vi "TalkToCVServer.vi"() -> ()   [LabVIEW 2019]
panel:
  out "Streaming":T1
  in  "Stop":bool
  out "Commands":T2(array[cluster])=[{"Info"={"version"="1.0", "Code"=200, "type"="text/html", "length"=-1}, "Header"="HTTP/1.0 200 OK\r\nServer: BaseHTTP/0.6 Python/3.7.2\r\nDate: Mon, 07 Dec 2020 21:12:43 GMT\r\nContent-type: text/html\r\n\r\n", "Body"="<html><head><title>Rogers Camera Code</title></head>\n                        <body><p>Rogers Camera  (192.168.86.35)<br>Camera Status: not connected</p>\n                        <a href = \"http://192.168.86.35:8000/settings\">Current Settings</a><br>\n                        <a href = \"http://192.168.86.35:8000/init\">Initialize Camera</a><br>\n                        <a href = \"http://192.168.86.35:8000/snap\">Snap an Image</a><br>\n                        <a href = \"http://192.168.86.35:8000/grab\">Stream Images</a><br>\n                        <a href = \"http://192.168.86.35:8000/close\">Close Camera Connection</a><br><br><br>\n                        <form action=\"/settings\"> \n                        <label for=\"camera\">Camera:</label>  \n                        <input type=\"number\" id=\"camera\" name=\"camera\" value=\"1\"><br> \n                        <label for=\"scale\">Scale Percent:</label>  \n                        <input type=\"number\" id=\"scale\" name=\"scale\" value=\"20\"><br>  \n                        <label for=\"rotate\">Orientation:</label> \n                        <select name=\"rotate\" id=\"rotate\" value=\"-1\"> \n                          <option value=\"-1\">no rotation</option> \n                          <option value=\"0\">90 CW</option> \n                          <option value=\"1\">180</option> \n                          <option value=\"2\">90 CCW</option> \n                        </select> <br><br>\n                        <input type=\"submit\" value=\"Update\">  \n                    </form><hr><p>Executing command: /</p></body></html>\r\n", "2D Picture"=bytes[494]}, {"Info"={"version"="1.0", "Code"=200, "type"="text/html", "length"=-1}, "Header"="HTTP/1.0 200 OK\r\nServer: BaseHTTP/0.6 Python/3.7.2\r\nDate: Mon, 07 Dec 2020 21:12:44 GMT\r\nContent-type: text/html\r\n\r\n", "Body"="<html><head><title>Rogers Camera Code</title></head>\n                        <body><p>Rogers Camera  (192.168.86.35)<br>Camera Status: not connected</p>\n                        <a href = \"http://192.168.86.35:8000/settings\">Current Settings</a><br>\n                        <a href = \"http://192.168.86.35:8000/init\">Initialize Camera</a><br>\n                        <a href = \"http://192.168.86.35:8000/snap\">Snap an Image</a><br>\n                        <a href = \"http://192.168.86.35:8000/grab\">Stream Images</a><br>\n                        <a href = \"http://192.168.86.35:8000/close\">Close Camera Connection</a><br><br><br>\n                        <form action=\"/settings\"> \n                        <label for=\"camera\">Camera:</label>  \n                        <input type=\"number\" id=\"camera\" name=\"camera\" value=\"1\"><br> \n                        <label for=\"scale\">Scale Percent:</label>  \n                        <input type=\"number\" id=\"scale\" name=\"scale\" value=\"40\"><br>  \n                        <label for=\"rotate\">Orientation:</label> \n                        <select name=\"rotate\" id=\"rotate\" value=\"-1\"> \n                          <option value=\"-1\">no rotation</option> \n                          <option value=\"0\">90 CW</option> \n                          <option value=\"1\">180</option> \n                          <option value=\"2\">90 CCW</option> \n                        </select> <br><br>\n                        <input type=\"submit\" value=\"Update\">  \n                    </form><hr><p>Executing command: /settings?camera=1&rotation=-1&scale=40</p>Settings:<br>Camera = 1<br>scaling = 40<br>Rotation = -1</body></html>\r\n", "2D Picture"=bytes[580]}, {"Info"={"version"="1.0", "Code"=200, "type"="text/html", "length"=-1}, "Header"="HTTP/1.0 200 OK\r\nServer: BaseHTTP/0.6 Python/3.7.2\r\nDate: Mon, 07 Dec 2020 21:12:44 GMT\r\nContent-type: text/html\r\n\r\n", "Body"="<html><head><title>Rogers Camera Code</title></head>\n                        <body><p>Rogers Camera  (192.168.86.35)<br>Camera Status: connected</p>\n                        <a href = \"http://192.168.86.35:8000/settings\">Current Settings</a><br>\n                        <a href = \"http://192.168.86.35:8000/init\">Initialize Camera</a><br>\n                        <a href = \"http://192.168.86.35:8000/snap\">Snap an Image</a><br>\n                        <a href = \"http://192.168.86.35:8000/grab\">Stream Images</a><br>\n                        <a href = \"http://192.168.86.35:8000/close\">Close Camera Connection</a><br><br><br>\n                        <form action=\"/settings\"> \n                        <label for=\"camera\">Camera:</label>  \n                        <input type=\"number\" id=\"camera\" name=\"camera\" value=\"1\"><br> \n                        <label for=\"scale\">Scale Percent:</label>  \n                        <input type=\"number\" id=\"scale\" name=\"scale\" value=\"40\"><br>  \n                        <label for=\"rotate\">Orientation:</label> \n                        <select name=\"rotate\" id=\"rotate\" value=\"-1\"> \n                          <option value=\"-1\">no rotation</option> \n                          <option value=\"0\">90 CW</option> \n                          <option value=\"1\">180</option> \n                          <option value=\"2\">90 CCW</option> \n                        </select> <br><br>\n                        <input type=\"submit\" value=\"Update\">  \n                    </form><hr><p>Executing command: /init</p>initializing camera # 1</body></html>\r\n", "2D Picture"=bytes[518]}, {"Info"={"version"="1.0", "Code"=200, "type"="text/html", "length"=-1}, "Header"="HTTP/1.0 200 OK\r\nServer: BaseHTTP/0.6 Python/3.7.2\r\nDate: Mon, 07 Dec 2020 21:12:45 GMT\r\nContent-type: text/html\r\n\r\n", "Body"="<html><head><title>Rogers Camera Code</title></head>\n                        <body><p>Rogers Camera  (192.168.86.35)<br>Camera Status: connected</p>\n                        <a href = \"http://192.168.86.35:8000/settings\">Current Settings</a><br>\n                        <a href = \"http://192.168.86.35:8000/init\">Initialize Camera</a><br>\n                        <a href = \"http://192.168.86.35:8000/snap\">Snap an Image</a><br>\n                        <a href = \"http://192.168.86.35:8000/grab\">Stream Images</a><br>\n                        <a href = \"http://192.168.86.35:8000/close\">Close Camera Connection</a><br><br><br>\n                        <form action=\"/settings\"> \n                        <label for=\"camera\">Camera:</label>  \n                        <input type=\"number\" id=\"camera\" name=\"camera\" value=\"1\"><br> \n                        <label for=\"scale\">Scale Percent:</label>  \n                        <input type=\"number\" id=\"scale\" name=\"scale\" value=\"40\"><br>  \n                        <label for=\"rotate\">Orientation:</label> \n                        <select name=\"rotate\" id=\"rotate\" value=\"-1\"> \n                          <option value=\"-1\">no rotation</option> \n                          <option value=\"0\">90 CW</option> \n                          <option value=\"1\">180</option> \n                          <option value=\"2\">90 CCW</option> \n                        </select> <br><br>\n                        <input type=\"submit\" value=\"Update\">  \n                    </form><hr><p>Executing command: /snap</p>snapping from camera # 1<br><br><img src=\"http://192.168.86.35:8000/snap.jpg\"></body></html>\r\n", "2D Picture"=bytes[37460]}, {"Info"={"version"="1.0", "Code"=200, "type"="text/html", "length"=-1}, "Header"="HTTP/1.0 200 OK\r\nServer: BaseHTTP/0.6 Python/3.7.2\r\nDate: Mon, 07 Dec 2020 21:12:45 GMT\r\nContent-type: text/html\r\n\r\n", "Body"="<html><head><title>Rogers Camera Code</title></head>\n                        <body><p>Rogers Camera  (192.168.86.35)<br>Camera Status: connected</p>\n                        <a href = \"http://192.168.86.35:8000/settings\">Current Settings</a><br>\n                        <a href = \"http://192.168.86.35:8000/init\">Initialize Camera</a><br>\n                        <a href = \"http://192.168.86.35:8000/snap\">Snap an Image</a><br>\n                        <a href = \"http://192.168.86.35:8000/grab\">Stream Images</a><br>\n                        <a href = \"http://192.168.86.35:8000/close\">Close Camera Connection</a><br><br><br>\n                        <form action=\"/settings\"> \n                        <label for=\"camera\">Camera:</label>  \n                        <input type=\"number\" id=\"camera\" name=\"camera\" value=\"1\"><br> \n                        <label for=\"scale\">Scale Percent:</label>  \n                        <input type=\"number\" id=\"scale\" name=\"scale\" value=\"40\"><br>  \n                        <label for=\"rotate\">Orientation:</label> \n                        <select name=\"rotate\" id=\"rotate\" value=\"-1\"> \n                          <option value=\"-1\">no rotation</option> \n                          <option value=\"0\">90 CW</option> \n                          <option value=\"1\">180</option> \n                          <option value=\"2\">90 CCW</option> \n                        </select> <br><br>\n                        <input type=\"submit\" value=\"Update\">  \n                    </form><hr><p>Executing command: /bad</p>unsupported path</body></html>\r\n", "2D Picture"=bytes[510]}, {"Info"={"version"="1.0", "Code"=200, "type"="text/html", "length"=-1}, "Header"="HTTP/1.0 200 OK\r\nServer: BaseHTTP/0.6 Python/3.7.2\r\nDate: Mon, 07 Dec 2020 21:12:45 GMT\r\nContent-type: text/html\r\n\r\n", "Body"="<html><head><title>Rogers Camera Code</title></head>\n                        <body><p>Rogers Camera  (192.168.86.35)<br>Camera Status: connected</p>\n                        <a href = \"http://192.168.86.35:8000/settings\">Current Settings</a><br>\n                        <a href = \"http://192.168.86.35:8000/init\">Initialize Camera</a><br>\n                        <a href = \"http://192.168.86.35:8000/snap\">Snap an Image</a><br>\n                        <a href = \"http://192.168.86.35:8000/grab\">Stream Images</a><br>\n                        <a href = \"http://192.168.86.35:8000/close\">Close Camera Connection</a><br><br><br>\n                        <form action=\"/settings\"> \n                        <label for=\"camera\">Camera:</label>  \n                        <input type=\"number\" id=\"camera\" name=\"camera\" value=\"1\"><br> \n                        <label for=\"scale\">Scale Percent:</label>  \n                        <input type=\"number\" id=\"scale\" name=\"scale\" value=\"40\"><br>  \n                        <label for=\"rotate\">Orientation:</label> \n                        <select name=\"rotate\" id=\"rotate\" value=\"-1\"> \n                          <option value=\"-1\">no rotation</option> \n                          <option value=\"0\">90 CW</option> \n                          <option value=\"1\">180</option> \n                          <option value=\"2\">90 CCW</option> \n                        </select> <br><br>\n                        <input type=\"submit\" value=\"Update\">  \n                    </form><hr><p>Executing command: /settings</p>Settings:<br>Camera = 1<br>scaling = 40<br>Rotation = -1</body></html>\r\n", "2D Picture"=bytes[546]}, {"Info"={"version"="error", "Code"=0, "type"="image/jpeg", "length"=3460}, "Header"="--jpgboundary\r\nContent-type: image/jpeg\r\nContent-length: 3460\r\n\r\n", "Body"="ÿØÿà\u0000\u0010JFIF\u0000\u0001\u0001\u0000\u0000\u0001\u0000\u0001\u0000\u0000ÿÛ\u0000C\u0000\u0002\u0001\u0001\u0001\u0001\u0001\u0002\u0001\u0001\u0001\u0002\u0002\u0002\u0002\u0002\u0004\u0003\u0002\u0002\u0002\u0002\u0005\u0004\u0004\u0003\u0004\u0006\u0005\u0006\u0006\u0006\u0005\u0006\u0006\u0006\u0007\t\b\u0006\u0007\t\u0007\u0006\u0006\b\u000b\b\t\n\n\n\n\n\u0006\b\u000b\f\u000b\n\f\t\n\n\nÿÛ\u0000C\u0001\u0002\u0002\u0002\u0002\u0002\u0002\u0005\u0003\u0003\u0005\n\u0007\u0006\u0007\n\n\n\n\n\n\n\n\n\n\n\n\n\n\n\n\n\n\n\n\n\n\n\n\n\n\n\n\n\n\n\n\n\n\n\n\n\n\n\n\n\n\n\n\n\n\n\n\n\nÿÀ\u0000\u0011\b\u0000`\u0000\u0003\u0001\"\u0000\u0002\u0011\u0001\u0003\u0011\u0001ÿÄ\u0000\u001f\u0000\u0000\u0001\u0005\u0001\u0001\u0001\u0001\u0001\u0001\u0000\u0000\u0000\u0000\u0000\u0000\u0000\u0000\u0001\u0002\u0003\u0004\u0005\u0006\u0007\b\t\n\u000bÿÄ\u0000µ\u0010\u0000\u0002\u0001\u0003\u0003\u0002\u0004\u0003\u0005\u0005\u0004\u0004\u0000\u0000\u0001}\u0001\u0002\u0003\u0000\u0004\u0011\u0005\u0012!1A\u0006\u0013Qa\u0007\"q\u00142¡\b#B±Á\u0015RÑð$3br\t\n\u0016\u0017\u0018\u0019\u001a%&'()*456789:CDEFGHIJSTUVWXYZcdefghijstuvwxyz¢£¤¥¦§¨©ª²³´µ¶·¸¹ºÂÃÄÅÆÇÈÉÊÒÓÔÕÖ×ØÙÚáâãäåæçèéêñòóôõö÷øùúÿÄ\u0000\u001f\u0001\u0000\u0003\u0001\u0001\u0001\u0001\u0001\u0001\u0001\u0001\u0001\u0000\u0000\u0000\u0000\u0000\u0000\u0001\u0002\u0003\u0004\u0005\u0006\u0007\b\t\n\u000bÿÄ\u0000µ\u0011\u0000\u0002\u0001\u0002\u0004\u0004\u0003\u0004\u0007\u0005\u0004\u0004\u0000\u0001\u0002w\u0000\u0001\u0002\u0003\u0011\u0004\u0005!1\u0006\u0012AQ\u0007aq\u0013\"2\b\u0014B¡±Á\t#3Rð\u0015brÑ\n\u0016$4á%ñ\u0017\u0018\u0019\u001a&'()*56789:CDEFGHIJSTUVWXYZcdefghijstuvwxyz¢£¤¥¦§¨©ª²³´µ¶·¸¹ºÂÃÄÅÆÇÈÉÊÒÓÔÕÖ×ØÙÚâãäåæçèéê...", "2D Picture"=bytes[36894]}, {"Info"={"version"="1.0", "Code"=200, "type"="text/html", "length"=-1}, "Header"="HTTP/1.0 200 OK\r\nServer: BaseHTTP/0.6 Python/3.7.2\r\nDate: Mon, 07 Dec 2020 21:12:48 GMT\r\nContent-type: text/html\r\n\r\n", "Body"="<html><head><title>Rogers Camera Code</title></head>\n                        <body><p>Rogers Camera  (192.168.86.35)<br>Camera Status: not connected</p>\n                        <a href = \"http://192.168.86.35:8000/settings\">Current Settings</a><br>\n                        <a href = \"http://192.168.86.35:8000/init\">Initialize Camera</a><br>\n                        <a href = \"http://192.168.86.35:8000/snap\">Snap an Image</a><br>\n                        <a href = \"http://192.168.86.35:8000/grab\">Stream Images</a><br>\n                        <a href = \"http://192.168.86.35:8000/close\">Close Camera Connection</a><br><br><br>\n                        <form action=\"/settings\"> \n                        <label for=\"camera\">Camera:</label>  \n                        <input type=\"number\" id=\"camera\" name=\"camera\" value=\"1\"><br> \n                        <label for=\"scale\">Scale Percent:</label>  \n                        <input type=\"number\" id=\"scale\" name=\"scale\" value=\"40\"><br>  \n                        <label for=\"rotate\">Orientation:</label> \n                        <select name=\"rotate\" id=\"rotate\" value=\"-1\"> \n                          <option value=\"-1\">no rotation</option> \n                          <option value=\"0\">90 CW</option> \n                          <option value=\"1\">180</option> \n                          <option value=\"2\">90 CCW</option> \n                        </select> <br><br>\n                        <input type=\"submit\" value=\"Update\">  \n                    </form><hr><p>Executing command: /close</p>closing camera # 1</body></html>\r\n", "2D Picture"=bytes[518]}]
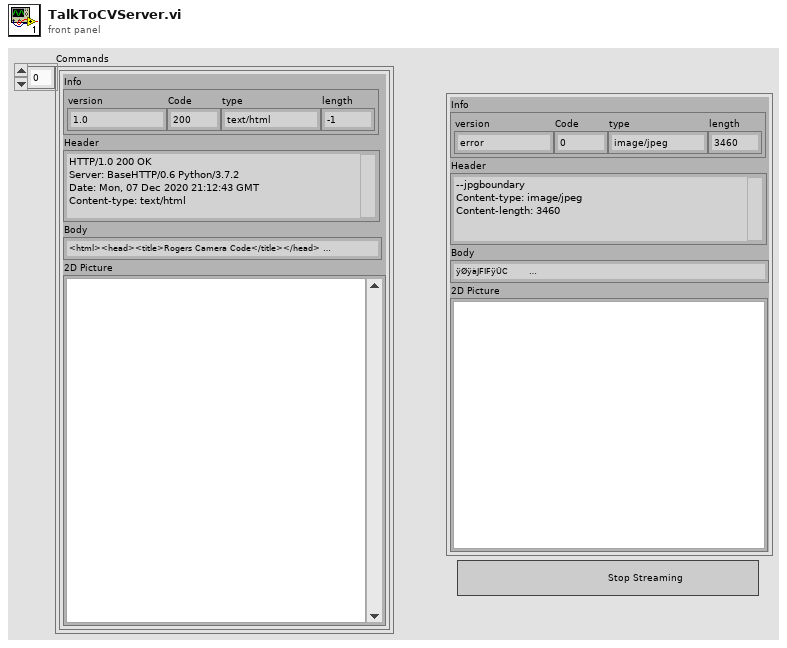
[diagram p1: front panel]
types:
  T1 = cluster{"Info":cluster{"version":string, "Code":i32, "type":string, "length":i32}, "Header":string, "Body":string, "2D Picture":picture}
  T2 = cluster{"Info":cluster{"version":string, "Code":i32, "type":string, "length":i32}, "Header":string, "Body":string, "2D Picture":picture}[]
  T3 = cluster{"Info":cluster{"version":string, "Code":i32, "type":string, "length":i32}, "Header":string, "Body":string}
  T4 = cluster{"version":string, "Code":i32, "type":string, "length":i32}
  T5 = cluster{"Info":cluster{"version":string, "Code":i32, "type":string, "length":i32}, "Header":string, "Body":string, "new picture":picture}
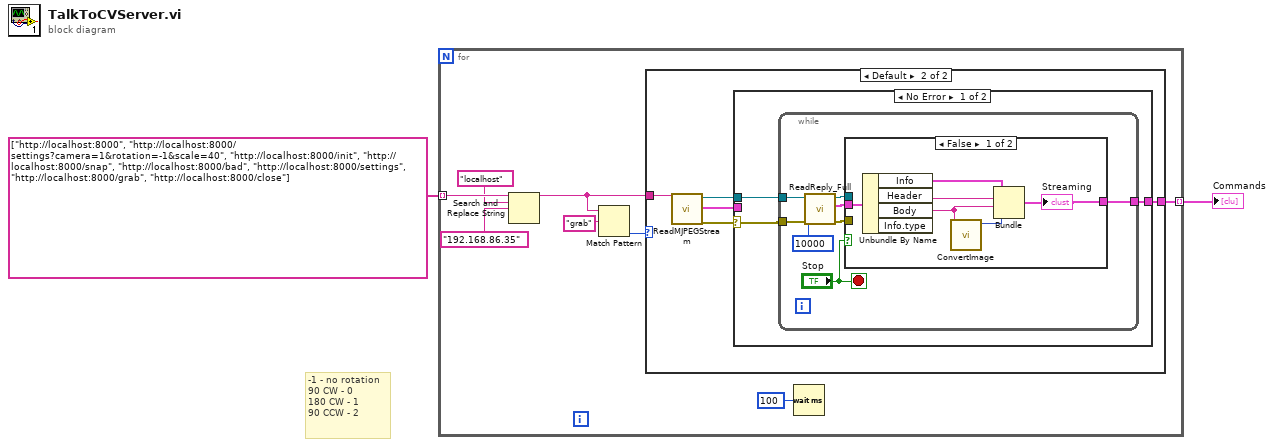
[diagram p0: block diagram]
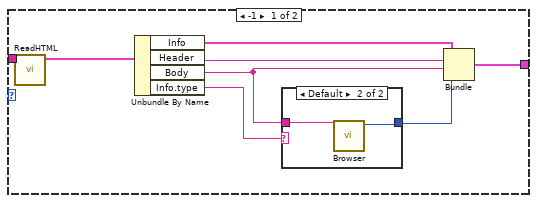
[diagram p2: hidden frame]
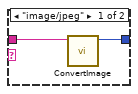
[diagram p3: hidden frame]
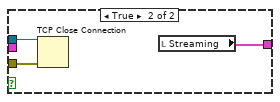
[diagram p4: hidden frame]
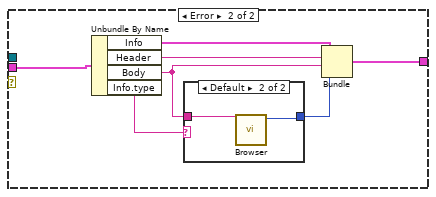
[diagram p5: hidden frame]
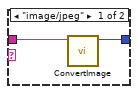
[diagram p6: hidden frame]
diagram:
  # "-1 - no rotation\n90 CW - 0\n180 CW - 1\n90 CCW - 2"
  n1 = for {
    tunnel: string[] ["http://localhost:8000", "http://localhost:8000/settings?camera=1&rotation=-1&scale=40", "http://localhost:8000/init", "http://localhost:8000/snap", "http://localhost:8000/bad", "http://localhost:8000/settings", "http://localhost:8000/grab", "http://localhost:8000/close"] -> [w6] mode=indexing
    tunnel: [w9] -> w1 mode=indexing
    n2 = Search and Replace String(input string=w6, search string="localhost", replace string="192.168.86.35" ("search string")) -> (result string=w3:string)  [unwired: 5 in, 3 out]
    n3 = Match Pattern(string=w3, regular expression="grab") -> (offset past match=w7:i32)  [unwired: 1 in, 3 out]
    n4 = case shown="Default" w7 {
      tunnel: [w18 w27] -> w9
      tunnel: w3 -> [w12 w26]
      frame -1 {
        n5 = call "ReadHTML.vi"("url"=w12) -> ("Info"=w11:T3)  [unwired: 8 in, 2 out]
        n6 = Unbundle By Name(w11) -> ("Info"=w13:T4, "Header"=w16:string, "Body"=w15:string, "Info.type"=w14:string)
        n7 = case shown="Default" w14 {
          tunnel: w15 -> [w20 w22]
          tunnel: [w19 w21] -> w17
          frame "image/jpeg" {
            n8 = call "ConvertImage.vi"("body"=w20) -> ("new picture"=w19:picture)  [unwired: 9 in, 1 out]
          }
          frame Default {
            n9 = call "Browser.vi"("html"=w22) -> ("2D Picture"=w21:picture)  [unwired: 10 in]
          }
        }
        n10 = Bundle("Info"=w13, "Header"=w16, "Body"=w15, "2D Picture"=w17) -> (w18:T1)  [unwired: 1 in]
      }
      frame Default {
        n11 = call "ReadMJPEGStream.vi"("url"=w26) -> ("error out"=w24:errorcluster, "Info"=w23:T3, "TCP out"=w25:refnum<k5>)  [unwired: 8 in]
        n12 = case shown="No Error" w24 {
          selector: w24 -> [w29 _]
          tunnel: [w30 w52] -> w27
          tunnel: w23 -> [_ w48]
          tunnel: w25 -> [w28 _]
          frame No Error {
            n13 = while {
              tunnel: [w38] -> w30
              tunnel: w29 -> [w37]
              tunnel: w28 -> [w31]
              stop <- "Stop" stop-if-true
              n14 = call "ReadReply_Full.vi"("error in (no error)"=w37, "timeout ms (60000)"=10000, "TCP in"=w31) -> ("error out"=w33:errorcluster, "Info"=w36:T3, "TCP out"=w34:refnum<k5>)  [unwired: 6 in]
              n15 = case shown="False" "Stop" {
                tunnel: [w40 w45] -> w38
                tunnel: w36 -> [w39 _]
                tunnel: w34 -> [_ w47]
                tunnel: w33 -> [_ w46]
                frame False {
                  n16 = Unbundle By Name(w39) -> ("Info"=w42:T4, "Header"=w44:string, "Body"=w43:string)  [unwired: 1 out]
                  n17 = call "ConvertImage.vi"("body"=w43) -> ("new picture"=w41:picture)  [unwired: 9 in, 1 out]
                  n18 = Bundle("Info"=w42, "Header"=w44, "Body"=w43, "new picture"=w41) -> (w40:T5)  [unwired: 1 in]
                  "Streaming" <- w40
                }
                frame True {
                  n19 = TCP Close Connection(connection ID=w47, error in (no error)=w46) -> ()  [unwired: 1 in, 2 out]
                  n20 = local read "Streaming"() -> (w45:T1)
                }
              }
            }
          }
          frame Error {
            n21 = Unbundle By Name(w48) -> ("Info"=w53:T4, "Header"=w54:string, "Body"=w50:string, "Info.type"=w51:string)
            n22 = case shown="Default" w51 {
              tunnel: w50 -> [w56 w58]
              tunnel: [w55 w57] -> w49
              frame "image/jpeg" {
                n23 = call "ConvertImage.vi"("body"=w56) -> ("new picture"=w55:picture)  [unwired: 9 in, 1 out]
              }
              frame Default {
                n24 = call "Browser.vi"("html"=w58) -> ("2D Picture"=w57:picture)  [unwired: 10 in]
              }
            }
            n25 = Bundle("Info"=w53, "Header"=w54, "Body"=w50, "2D Picture"=w49) -> (w52:T1)  [unwired: 1 in]
          }
        }
      }
    }
    n26 = Wait (ms)(milliseconds to wait=u32 100) -> ()  [unwired: 1 out]
  }
  "Commands" <- w1
